vi "Multiline_string_to_array.vi"(11 "Input string":string) -> (2 "Token positions":i32[](array[numeric]), 3 "String Array Out":string[](array[string]), 4 "LF found?":bool, 5 "Number of LF matches":i32)   [LabVIEW 2019]
uses:
  <vilib>/regexp/Match Regular Expression.xnode
panel:
  out "Str arr lengths":i32[](array[numeric])
  out "Token positions":i32[](array[numeric])
  out "String Array Out 2":string[](array[string])
  out "Substring before match array":string[](array[string])
  out "Input string length":i32
  out "offset past token":i32
  out "substring before match":string
  # "cmd.exe                    17160 Console                 0      3,196 K Running         GS66-BAMXP2\\shutters"
  # "Old programming/obsolete? (While loop at the bottom)"
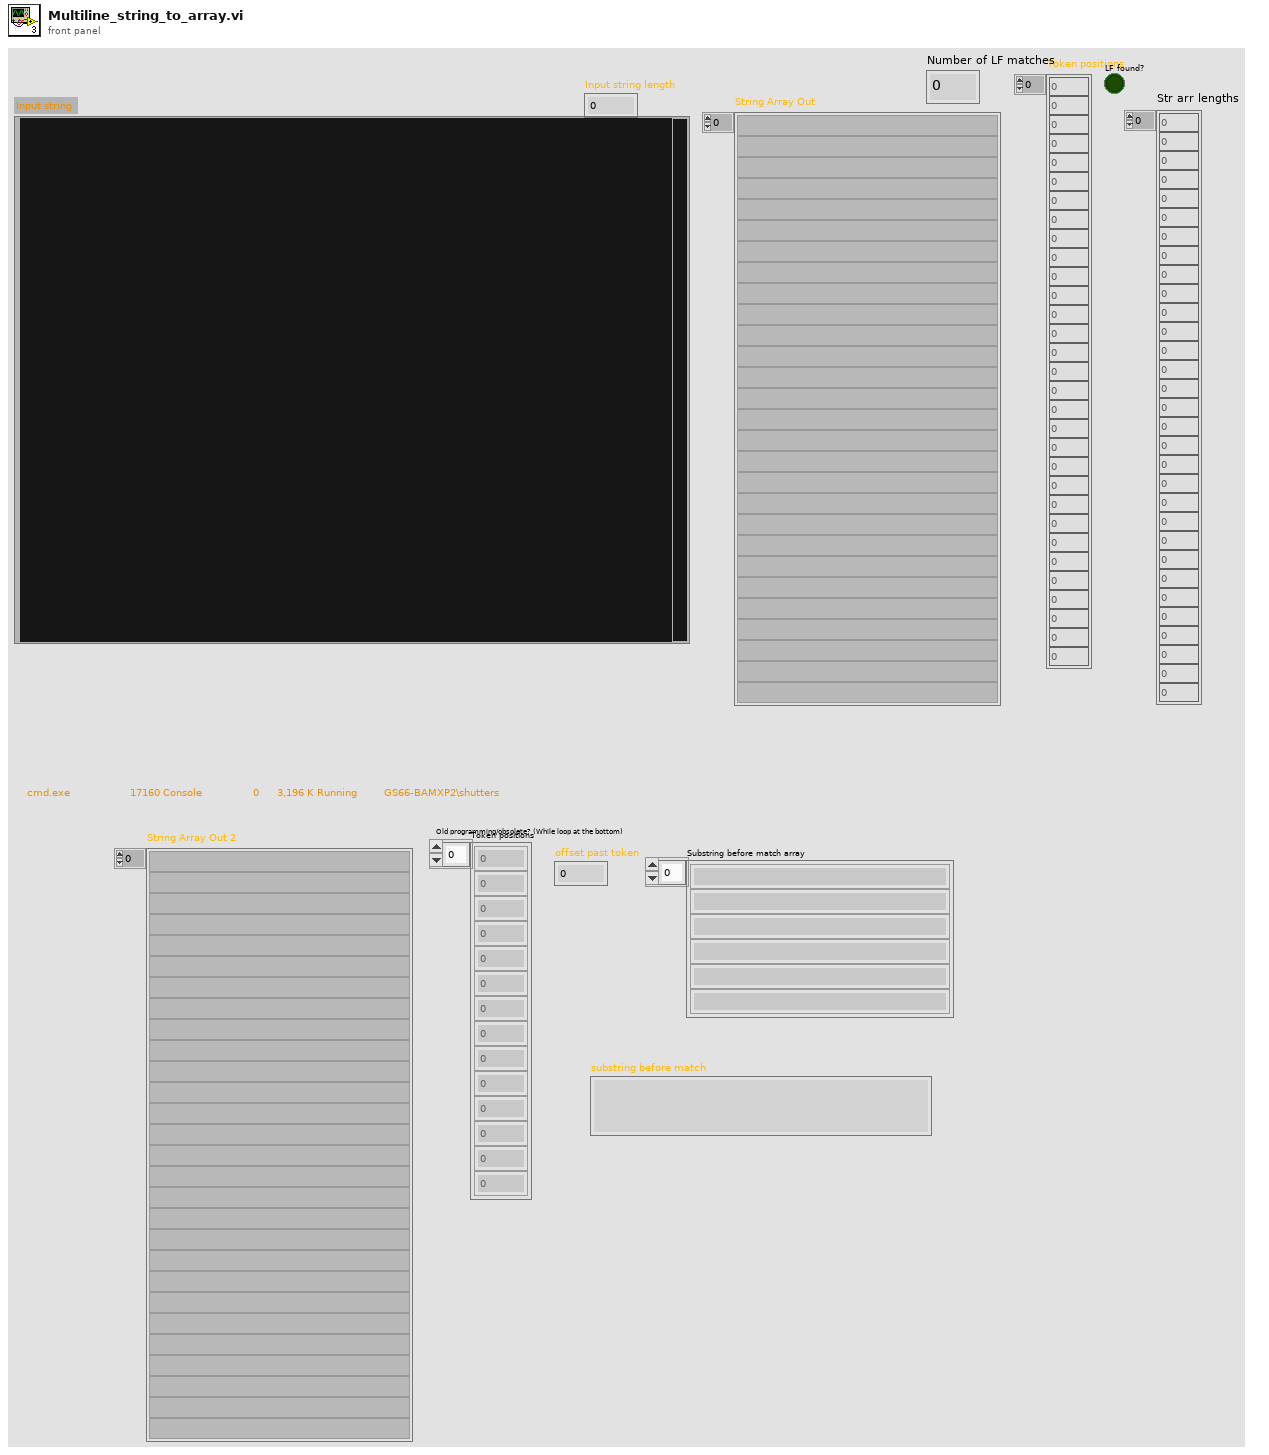
[diagram p1: front panel]
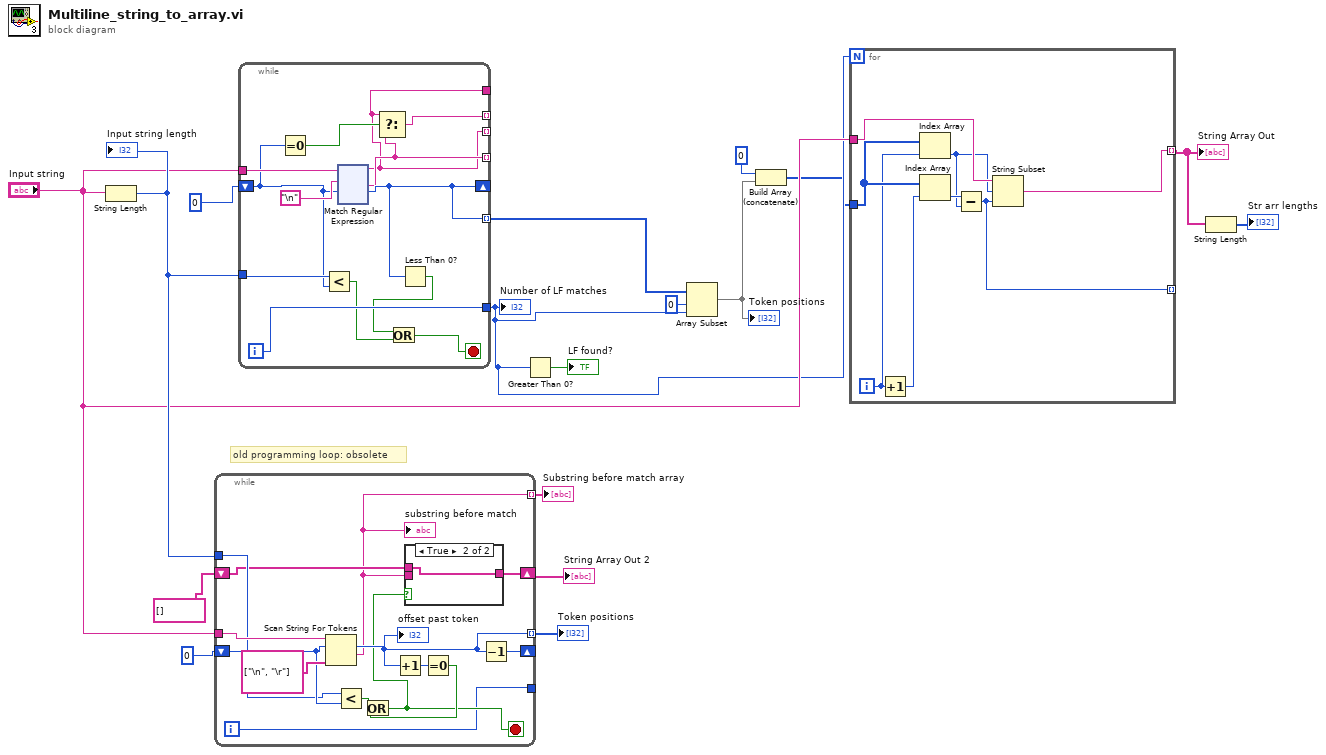
[diagram p0: block diagram]
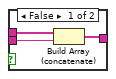
[diagram p2: hidden frame]
diagram:
  # "old programming loop: obsolete"
  n1 = String Length(string="Input string") -> (length=w13:i32)
  "Input string length" <- w13
  n2 = while {
    tunnel: w13 -> [w28]
    shift-right: [w19] -> _
    shift-left: 0 ("offset past token") -> [w29]
    tunnel: "Input string" -> [w31]
    tunnel: [w24] -> w11 mode=indexing
    shift-right: [w23] -> w12
    shift-left: string[] [] -> [w22]
    tunnel: [w20] -> w15 mode=indexing
    tunnel: [w18] -> _
    i -> [w18]
    stop <- w21 stop-if-true
    n3 = Scan String For Tokens(6:string[] ["\n", "\r"] ("delimiters (\\s,\\t,\\r,\\n)"), 8:w29, 9:w31) -> (1:w20:string, 2:w24:i32)  [unwired: 3 in, 2 out]
    "substring before match" <- w20
    "offset past token" <- w24
    n4 = Less?(x=w28, y=w29) -> (x < y?=w27:bool)
    n5 = Increment(x=w24) -> (x+1=w26:i32)
    n6 = Equal To 0?(x=w26) -> (x = 0?=w25:bool)
    n7 = Or(x=w27, y=w25) -> (x .or. y?=w21:bool)
    n8 = case shown="True" w21 {
      tunnel: w20 -> [w34 _]
      tunnel: [w33 w35] -> w23
      tunnel: w22 -> [w32 w35]
      frame False {
        n9 = Build Array (concatenate)(w32, w34) -> (w33:string[])
      }
      frame True {
      }
    }
    n10 = Decrement(x=w24) -> (x-1=w19:i32)
  }
  "Substring before match array" <- w15
  "String Array Out 2" <- w12
  "Token positions" <- w11
  n11 = while {
    tunnel: "Input string" -> [w48]
    shift-right: [w45] -> _
    shift-left: 0 ("offset past token") -> [w37]
    tunnel: [w44] -> _ mode=indexing
    tunnel: [w41] -> _ mode=indexing
    tunnel: [w46] -> w6
    tunnel: [w45] -> w10 mode=indexing
    tunnel: [w42] -> _ mode=indexing
    tunnel: [w41] -> _
    tunnel: w13 -> [w38]
    i -> [w46]
    stop <- w40 stop-if-true
    n12 = Equal To 0?(x=w37) -> (x = 0?=w43:bool)
    n13 = Less?(x=w38, y=w37) -> (x < y?=w36:bool)
    n14 = xnode "Match Regular Expression"("input string"=w48, "regular expression"="\n", "offset (0)"=w37) -> ("before match"=w41:string, "after match"=w44:string, "offset past match"=w45:i32)  [unwired: 3 in, 2 out]
    n15 = Select(t=w41, s=w43, f=w44) -> (s? t:f=w42:string)
    n16 = Less Than 0?(x=w45) -> (x < 0?=w39:bool)
    n17 = Or(x=w39, y=w36) -> (x .or. y?=w40:bool)
  }
  "Number of LF matches" <- w6
  n18 = Greater Than 0?(x=w6) -> (x > 0?=→"LF found?":bool)
  n19 = Array Subset(array=w10, index=0, length=w6) -> (w4:i32[])
  "Token positions" <- w4
  n20 = Build Array (concatenate)(0, w4) -> (w3:i32[])
  n21 = for {
    N: w6 -> [_]
    tunnel: "Input string" -> [w167]
    tunnel: w3 -> [w163]
    tunnel: [w165] -> w1 mode=indexing
    tunnel: [w161] -> _ mode=indexing
    i -> [w160]
    n22 = Increment(x=w160) -> (x+1=w162:i32)
    n23 = Index Array(array=w163, index=w160) -> (element=w164:i32)
    n24 = Index Array(array=w163, index=w162) -> (element=w166:i32)
    n25 = Subtract(x=w166, y=w164) -> (x-y=w161:i32)
    n26 = String Subset(string=w167, offset (0)=w164, length (rest)=w161) -> (substring=w165:string)
  }
  "String Array Out" <- w1
  n27 = String Length(string=w1) -> (length=→"Str arr lengths":i32[])
